vi "Read Comm to Main.vi"(8 "error in (no error)":errorcluster, 11 "CIFPlugin in":refnum<class "Template_Plugin.lvclass">) -> (0 "error out":errorcluster, 3 "CIFPlugin out":refnum<class "Template_Plugin.lvclass">)   [LabVIEW 2021, in "Template_Plugin.lvclass"]
uses:
  Template_Plugin.lvclass
  <vilib>/CIF Foundation/CIF CIPC/TypeDefs/Read Configuration.ctl
  <vilib>/CIF Foundation/CIF CIPC/TypeDefs/Read Position.ctl
  Common/Typedef/OOB Comm/To Main Command Payload.ctl
  Common/Typedef/OOB Comm/To Main Command.ctl
  Common/Typedef/OOB Comm/To Main Command Data.ctl
  Template_Plugin.lvclass/Template_Plugin.ctl
  4efb0375-f1de-4191-b03f-44d34e6646cb.vi
  525c214c-2a6b-4e7b-b3ce-0ad96b412d2f.vi
  <vilib>/CIF Foundation/CIF CIPC/SubVIs/Wait For N Elements Available.vi
  <vilib>/CIF Foundation/CIF CIPC/SubVIs/Check Error.vi
  <vilib>/CIF Foundation/CIF CIPC/SubVIs/Get dll Path.vi
  <vilib>/CIF Foundation/CIF CIPC/SubVIs/Get Element Read Position.vi
  <vilib>/CIF Foundation/CIF CIPC/SubVIs/Set Element Read Position.vi
  <vilib>/CIF Foundation/CIF CIPC/SubVIs/Get Element Info Variant.vi
  <vilib>/CIF Foundation/CIF CIPC/SubVIs/Check Error Core.vi
  Common/Template_Common.lvlib
  <vilib>/CIF Foundation/CIF CIPC/CIF_NI_CIPC.lvlib
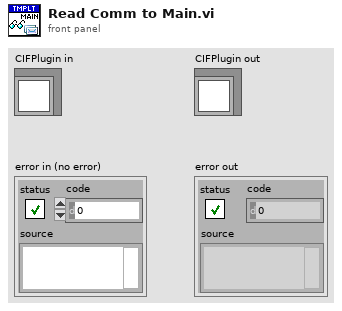
[diagram p1: front panel]
types:
  T1 = typedef "CIF_NI_CIPC.lvlib/Read Configuration.ctl" = cluster{"Read Position":T2, "Element Offset":i32, "Prepend Array Size":bool, "Get Read Position":bool}
  T2 = typedef "CIF_NI_CIPC.lvlib/Read Position.ctl" = enum8{"Next", "Newest", "Oldest", "Next Available", "Absolute"}
  T3 = typedef "Template_Common.lvlib/To Main Command Payload.ctl" = cluster{"Command":T4, "-> Main":T5}
  T4 = typedef "Template_Common.lvlib/To Main Command.ctl" = enum8{"Read Data", "Read DVR Data"}
  T5 = typedef "Template_Common.lvlib/To Main Command Data.ctl" = cluster{"Cmd Data 1 -> Main":i16}
  T6 = typedef "Template_Common.lvlib/To Main DVR Data.ctl" = cluster{"Data 1 DVR  -> Main":i32}
  T7 = typedef "Template_Common.lvlib/To Main Cyclic Data.ctl" = cluster{"Data 1 -> Main":i16}
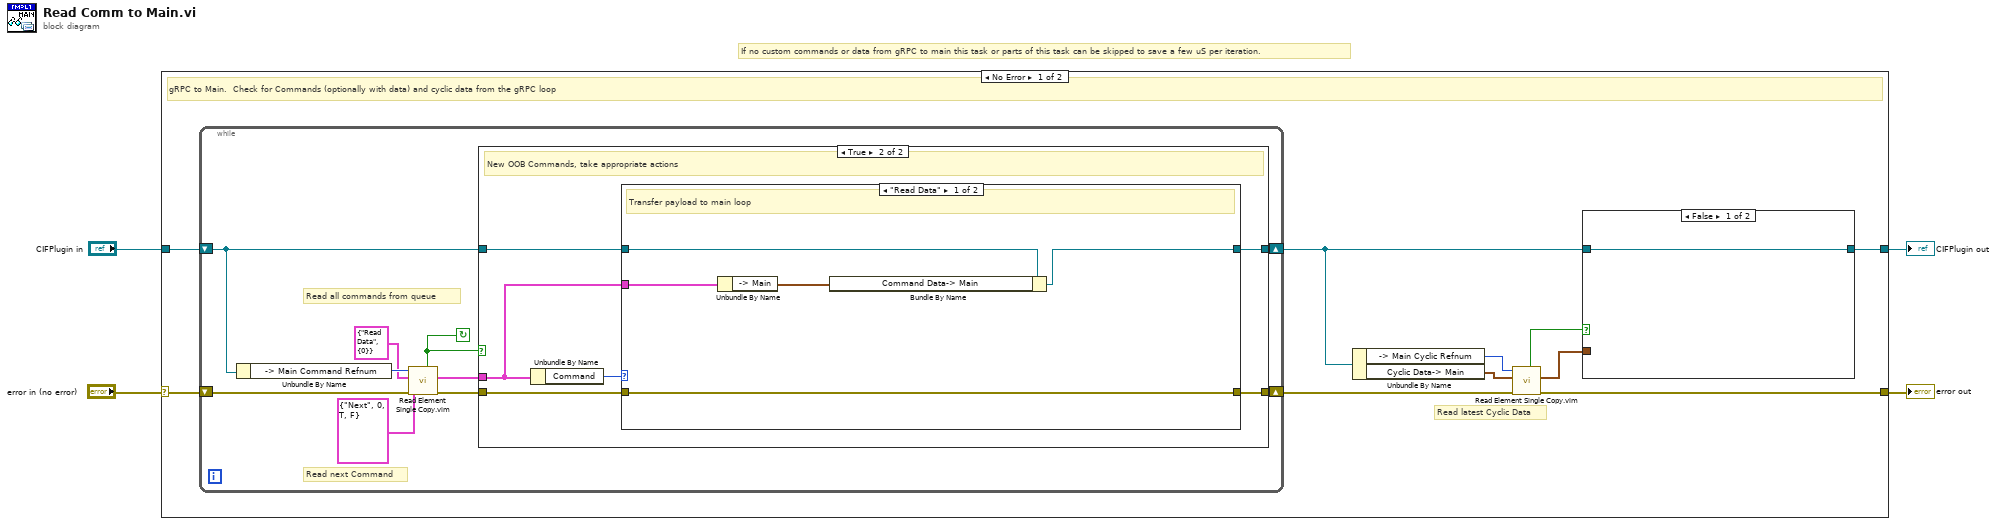
[diagram p0: block diagram]
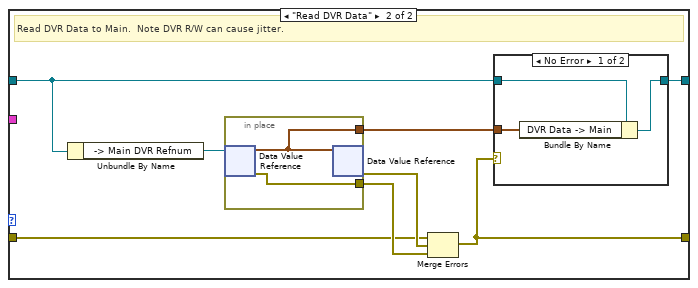
[diagram p3: hidden frame]
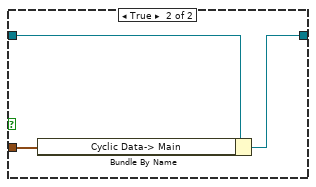
[diagram p5: hidden frame]
diagram:
  # "If no custom commands or data from gRPC to main this task or parts of this task can be skipped to save a few uS per iteration."
  n1 = case shown="No Error" "error in (no error)" {
    selector: "error in (no error)" -> [w14 w57]
    tunnel: [w10 w57] -> w3
    tunnel: [w5 w56] -> w1
    tunnel: "CIFPlugin in" -> [w13 w56]
    frame No Error {
      # "Read latest Cyclic Data"
      # "gRPC to Main.  Check for Commands (optionally with data) and cyclic data from the gRPC loop"
      n2 = while {
        shift-right: [w18] -> w11
        shift-left: w14 -> [w23]
        shift-right: [w16] -> w6
        shift-left: w13 -> [w22]
        stop <- w15 continue-if-true
        # "Read all commands from queue"
        # "Read next Command"
        n3 = Unbundle By Name(w22) -> ("-> Main Command Refnum"=w24:u64)
        n4 = call "Read Element Single Copy.vim"("error in (no error)"=w23, "Read Configuration"=T1 {"Read Position"=enum."Next", "Element Offset"=0, "Prepend Array Size"=TRUE, "Get Read Position"=FALSE}, "Data in"=T3 {"Command"=enum."Read Data", "-> Main"={"Cmd Data 1 -> Main"=0}} ("Payload"), "CIPC Reference in"=w24) -> ("error out"=w20:errorcluster, "Data out"=w19:T3, "Success"=w15:bool)  [unwired: 3 in, 2 out]
        n5 = case shown="True" w15 {
          tunnel: w22 -> [w26 w32]
          tunnel: [w26 w27] -> w16
          tunnel: w20 -> [w25 w31]
          tunnel: [w25 w30] -> w18
          tunnel: w19 -> [_ w28]
          frame False {
            # "No new OOB Commands"
          }
          frame True {
            # "New OOB Commands, take appropriate actions"
            n6 = Unbundle By Name(w28) -> ("Command"=w29:T4)
            n7 = case shown="\"Read Data\"" w29 {
              tunnel: w31 -> [w37 w41]
              tunnel: w32 -> [w35 w40]
              tunnel: [w37 w38] -> w30
              tunnel: w28 -> [w36 _]
              tunnel: [w33 w39] -> w27
              frame "Read Data" {
                # "Transfer payload to main loop"
                n8 = Unbundle By Name(w36) -> ("-> Main"=w34:T5)
                n9 = Bundle By Name(cluster=w35, "Command Data-> Main"=w34) -> (w33:refnum<class "Template_Plugin.lvclass">)
              }
              frame "Read DVR Data" {
                # "Read DVR Data to Main.  Note DVR R/W can cause jitter."
                n10 = Unbundle By Name(w40) -> ("-> Main DVR Refnum"=w43:refnum<data-value>)
                n11 = in-place {
                  in-place-border: [w51] -> w45
                  in-place-border: [w50] -> w42
                  n12 = in-place-dvr #1(w43) -> (w50:T6, w51:errorcluster)
                  n13 = in-place-dvr #1(w50) -> (w44:errorcluster)  [unwired: 1 out]
                }
                n14 = Merge Errors(w41, w44, w45) -> (w38:errorcluster)
                n15 = case shown="No Error" w38 {
                  tunnel: w42 -> [w48 _]
                  tunnel: w40 -> [w47 w49]
                  tunnel: [w46 w49] -> w39
                  frame No Error {
                    n16 = Bundle By Name(cluster=w47, "DVR Data -> Main"=w48) -> (w46:refnum<class "Template_Plugin.lvclass">)
                  }
                  frame Error {
                  }
                }
              }
            }
          }
        }
      }
      n17 = Unbundle By Name(w6) -> ("-> Main Cyclic Refnum"=w12:u64, "Cyclic Data-> Main"=w9:T7)
      n18 = call "Read Element Single Copy.vim"("error in (no error)"=w11, "Data in"=w9, "CIPC Reference in"=w12) -> ("error out"=w10:errorcluster, "Data out"=w7:T7, "Success"=w8:bool)  [unwired: 4 in, 2 out]
      n19 = case shown="False" w8 {
        tunnel: w7 -> [_ w54]
        tunnel: w6 -> [w52 w55]
        tunnel: [w52 w53] -> w5
        frame False {
        }
        frame True {
          n20 = Bundle By Name(cluster=w55, "Cyclic Data-> Main"=w54) -> (w53:refnum<class "Template_Plugin.lvclass">)
        }
      }
    }
    frame Error {
    }
  }
  "error out" <- w3
  "CIFPlugin out" <- w1
